vi "Actor Core.vi"(8 "error in":errorcluster, 11 "UI in":refnum<class "UI.lvclass">) -> (0 "error out":errorcluster, 3 "Actor out":refnum<class "Actor.lvclass">)   [LabVIEW 2020, in "UI.lvlib" / "UI.lvclass"]
doc: "<p>(<strong>Filename</strong>: <span class=\"dnl\">Actor Framework.lvlib:Actor.lvclass:Actor Core.vi</span>)</p>\n<p>Receives messages to the actor, reacts to them, and initiates any error handling that may shut the actor down.</p>\n<p>Descendant classes may override this VI to append parallel tasks for the actor to complete while it handles messages. Overrides use the <a href=\"nihelplauncher://docs/csh?context=lvcore_glang_udclass\">Call Parent Class Method</a> node.</p>"
uses:
  UI.lvclass
  C:/Program Files/National Instruments/LabVIEW 2026/vi.lib/ActorFramework/Actor/Actor.lvclass
  <vilib>/ActorFramework/Actor/Actor.lvclass
  <vilib>/ActorFramework/Actor/Actor.lvclass/Actor.ctl
  <vilib>/ActorFramework/Message Enqueuer/Message Enqueuer.lvclass/Message Enqueuer.ctl
  UI.lvclass/UI.ctl
  Supervisor/Supervisor Messages/Start Acquisition Msg/Start Acquisition Msg.lvclass/Start Acquisition Msg.ctl
  Supervisor/Supervisor Messages/Stop Acquisition Msg/Stop Acquisition Msg.lvclass
  C:/Program Files/National Instruments/LabVIEW 2026/vi.lib/ActorFramework/Message/Message.lvclass
  Supervisor/Supervisor Messages/Start Acquisition Msg/Start Acquisition Msg.lvclass
  Supervisor/Supervisor Messages/Close UI Msg/Close UI Msg.lvclass
  <vilib>/ActorFramework/Message Enqueuer/Message Enqueuer.lvclass
  C:/Users/taacr/OneDrive/HP/Local/Actor Framework/UI/UI/UI.lvclass
panel:
  in  "Threshold":dbl
  out "DAQmx Digital Channel":tag
  in  "Button":bool
  out "Status":bool[](array[boolean])
  out "Waveform Graph":waveform(dbl)[](graph)
  out "DAQmx Analog Channel":tag
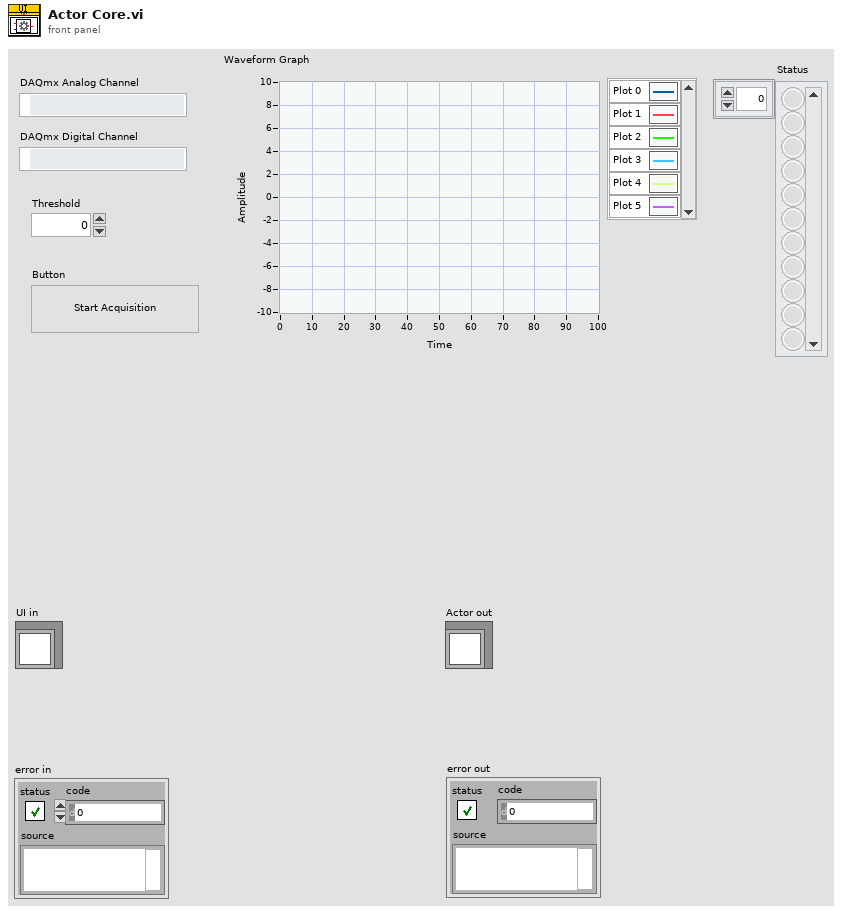
[diagram p1: front panel]
types:
  T1 = typedef "UI.lvlib/UI.lvclass/User Events.ctl" = cluster{"Stop Event":refnum<user-event>, "DAQmx Analog Channel Event":refnum<user-event>, "Waveform Graph Event":refnum<user-event>, "DAQmx Digital Channel":refnum<user-event>, "Status Event":refnum<user-event>, "Over Threshold Event":refnum<user-event>}
  T2 = enum8{"Enabled", "Disabled", "Disabled and Grayed Out"}
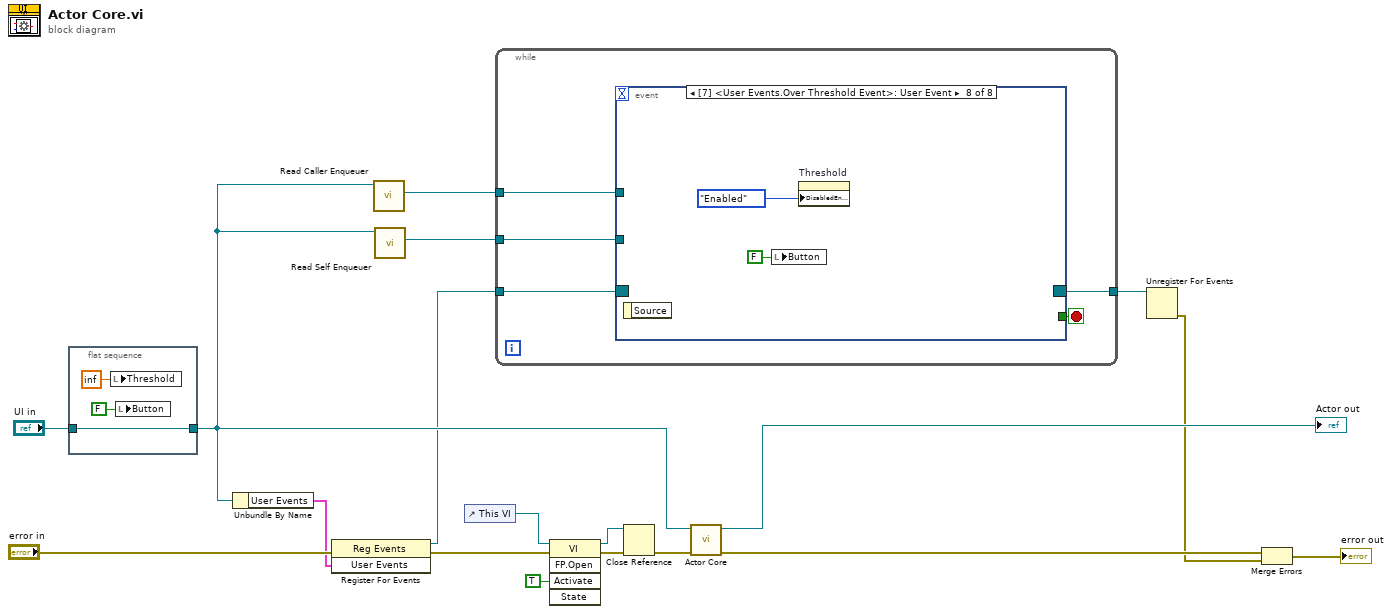
[diagram p0: block diagram]
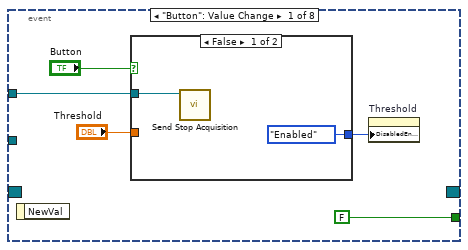
[diagram p2: hidden frame]
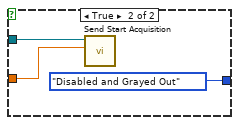
[diagram p3: hidden frame]
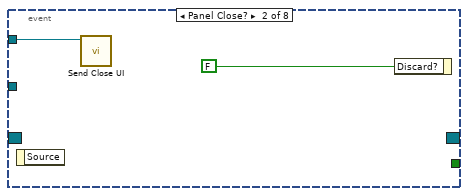
[diagram p4: hidden frame]
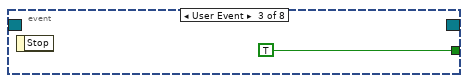
[diagram p5: hidden frame]
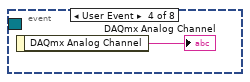
[diagram p6: hidden frame]
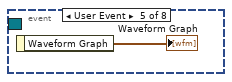
[diagram p7: hidden frame]
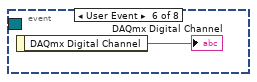
[diagram p8: hidden frame]
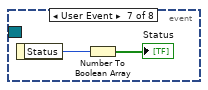
[diagram p9: hidden frame]
diagram:
  n1 = flat-sequence {
    tunnel: [w20] -> w10
    tunnel: "UI in" -> [w20]
    frame #0 {
      n2 = local write "Threshold"(inf ("Threshold")) -> ()
      n3 = local write "Button"(FALSE ("Button")) -> ()
    }
  }
  n4 = Unbundle By Name(w10) -> ("User Events"=w8:T1)
  n5 = register-events(error in="error in", w8) -> (reference out=w7:refnum<event-registration>, error out=w6:errorcluster)  [unwired: 1 in]
  n6 = call <vilib>:"Read Caller Enqueuer.vi"("Actor"=w10) -> ("Caller Enqueuer"=w17:refnum<class "Message Enqueuer.lvclass">)  [unwired: 10 in]
  n7 = call <vilib>:"Read Self Enqueuer.vi"("Actor"=w10) -> ("Self Enqueuer"=w16:refnum<class "Message Enqueuer.lvclass">)  [unwired: 10 in]
  n8 = control-ref of="This VI"() -> (w5:refnum<vi>)
  n9 = while {
    tunnel: w17 -> [w26]
    tunnel: w16 -> [w25]
    tunnel: [w24] -> w15
    tunnel: w7 -> [w22]
    stop <- w23 stop-if-true
    n10 = event shown="[7] <User Events.Over Threshold Event>: User Event" {
      selector: w22 -> [_ _ _ _ _ _ _ _]
      dyn-events: [_ _ _ _ _ _ _ _] -> w24
      timeout: _ -> [_ _ _ _ _ _ _ _]
      tunnel: w26 -> [w30 w37 _ _ _ _ _ _]
      tunnel: w25 -> [_ _ _ _ _ _ _ _]
      tunnel: [FALSE _ TRUE _ _ _ _ _] -> w23
      event "Button": Value Change {
        n11 = event-data() -> ()  [unwired: 1 in, 1 out]
        n12 = case shown="False" "Button" {
          tunnel: w30 -> [w33 w36]
          tunnel: "Threshold" -> [_ w35]
          tunnel: [T2."Enabled" ("DisabledEnum") T2."Disabled and Grayed Out" ("DisabledEnum")] -> w27
          frame False {
            n13 = call "Send Stop Acquisition.vi"("Message Enqueuer"=w33) -> ()  [unwired: 9 in, 2 out]
          }
          frame True {
            n14 = call "Send Start Acquisition.vi"("Threshold"=w35, "Message Enqueuer"=w36) -> ()  [unwired: 8 in, 2 out]
          }
        }
        n15 = property on="Threshold" class="DigNum (strict)"("DisabledEnum"=w27) -> ()  [unwired: 2 in, 2 out]
      }
      event Panel Close? {
        n16 = event-data() -> ()  [unwired: 1 in, 1 out]
        n17 = call "Send Close UI.vi"("Message Enqueuer"=w37) -> ()  [unwired: 9 in, 2 out]
        n18 = event-data("Discard?"=FALSE) -> ()  [unwired: 1 in, 1 out]
      }
      event User Event {
        n19 = event-data() -> ()  [unwired: 1 in, 1 out]
      }
      event User Event {
        n20 = event-data() -> ("DAQmx Analog Channel"=→"DAQmx Analog Channel":tag)  [unwired: 1 in]
      }
      event User Event {
        n21 = event-data() -> ("Waveform Graph"=→"Waveform Graph":waveform(dbl)[])  [unwired: 1 in]
      }
      event User Event {
        n22 = event-data() -> ("DAQmx Digital Channel"=→"DAQmx Digital Channel":tag)  [unwired: 1 in]
      }
      event User Event {
        n23 = event-data() -> ("Status"=w44:u8)  [unwired: 1 in]
        n24 = Number To Boolean Array(number=w44) -> (Boolean array=→"Status":bool[])
      }
      event User Event {
        n25 = event-data() -> ()  [unwired: 1 in, 1 out]
        n26 = local write "Button"(FALSE ("Button")) -> ()
        n27 = property on="Threshold" class="DigNum (strict)"("DisabledEnum"=T2."Enabled") -> ()  [unwired: 2 in, 2 out]
      }
    }
  }
  n28 = invoke class="VI" method="FP.Open"(reference=w5, error in=w6, "Activate"=TRUE ("Activate?")) -> (reference out=w3:refnum<vi>, error out=w4:errorcluster)  [unwired: 2 in, 3 out]
  n29 = Close Reference(reference=w3, error in (no error)=w4) -> (error out=w2:errorcluster)
  n30 = call-parent "Actor Core.vi"("error in"=w2, "Actor in"=w10) -> ("error out"=w14:errorcluster, "Actor out"=→"Actor out":refnum<class "Actor.lvclass">)  [unwired: 8 in]
  n31 = Unregister For Events(event registration refnum=w15) -> (error out=w13:errorcluster)  [unwired: 1 in]
  n32 = Merge Errors(w14, w13) -> (→"error out":errorcluster)
